vi "DefineTest.vi"(8 "error in":errorcluster) -> (0 "error out":errorcluster)   [LabVIEW 2016, in "Drona.lvlib"]
doc: "Defines the Test in Caraya Framework.\n\nAll assertions after calling this and present within the same block diagram, will become part of this test."
uses:
  Drona.lvlib
  <vilib>/addons/_JKI Toolkits/Caraya/classes/Test/Test.lvclass
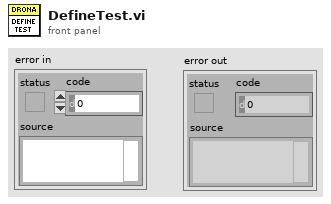
[diagram p1: front panel]
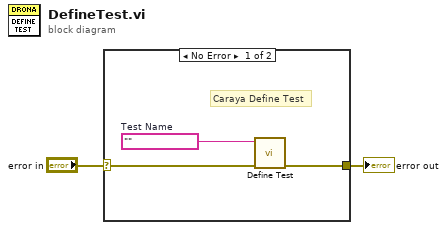
[diagram p0: block diagram]
diagram:
  n1 = case shown="No Error" "error in" {
    selector: "error in" -> [w4 w6]
    tunnel: [w3 w6] -> w1
    frame No Error {
      w5 = ""  # Test Name
      # "Caraya Define Test"
      n2 = call <vilib>:"Define Test.vi"("error in (no error)"=w4, "Label (VI Title)"=w5) -> ("error out"=w3:errorcluster)  [unwired: 8 in, 1 out]
    }
    frame Error {
    }
  }
  "error out" <- w1
